vi "Read Step Data (AC Parallel Program Mode).vi"   [LabVIEW 2016, in "APT 300XAC Series.lvlib"]
doc: "Reads the Step data from the instrument. AC Parallel Program Mode only."
uses:
  APT 300XAC Series.lvlib
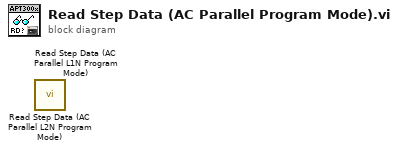
[diagram p0: block diagram]
diagram:
  n1 = call "Read Step Data (AC Parallel L2N Program Mode).vi"() -> ()  [unwired: 13 in, 3 out]
  n2 = call "Read Step Data (AC Parallel L1N Program Mode).vi"() -> ()  [unwired: 13 in, 3 out]
